vi "Generate Custom Error.vi"(8 "error in":errorcluster, 10 "PAR1":string, 11 "Enum":T1) -> (0 "error out":errorcluster)   [LabVIEW 2013, in "GOLPI library.lvlib"]
uses:
  GOLPI library.lvlib
  Custom Error Codes Enum Type Def.vi
  <vilib>/Utility/error.llb/Error Cluster From Error Code.vi
  <vilib>/ErrorRing/Error Ring.xnode
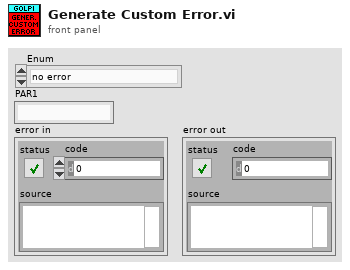
[diagram p1: front panel]
types:
  T1 = typedef "GOLPI library.lvlib/Custom Error Codes Enum Type Def.vi" = enum16{"no error", "00 working directory PAR1 missing", "01 octave binary PAR1 missing", "02 octave report error PAR1", "03 empty output last cmd PAR1", "04 missing temporary file PAR1", "10 var PAR1 not string", "11 var PAR1 not num, scal, ~compl", "12 var PAR1 not num, scal, compl", "13 var PAR1 not num, vect, ~compl", "14 var PAR1 not num, vect, compl", "15 var PAR1 not num, mat, ~compl", "16 var PAR1 not num, mat, ~compl", "99 not finished"}
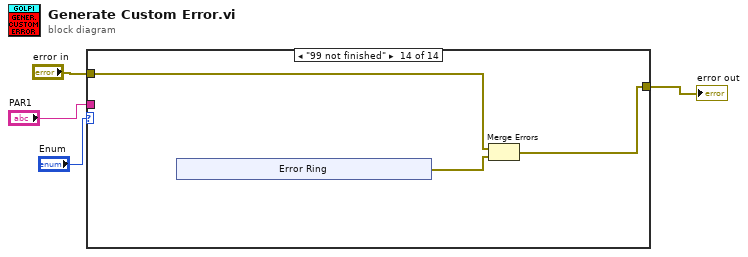
[diagram p0: block diagram]
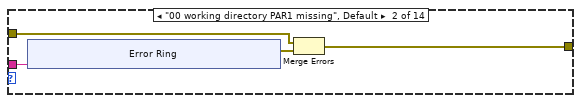
[diagram p3: hidden frame]
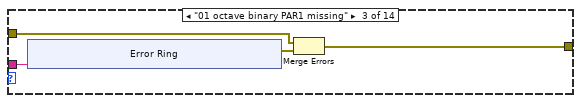
[diagram p4: hidden frame]
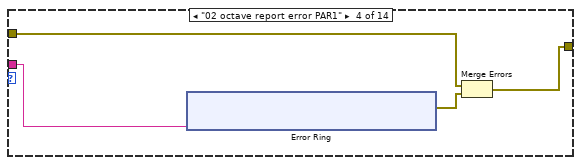
[diagram p5: hidden frame]
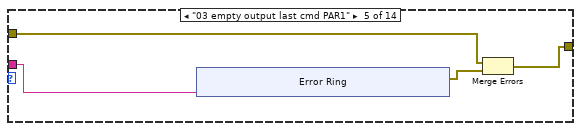
[diagram p6: hidden frame]
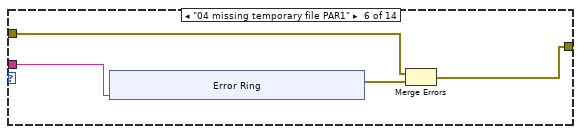
[diagram p7: hidden frame]
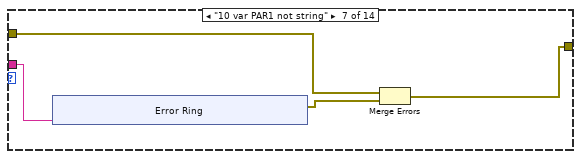
[diagram p8: hidden frame]
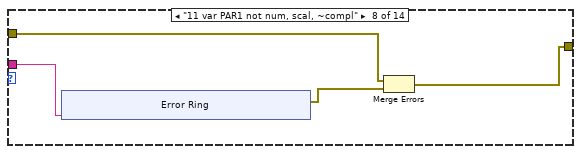
[diagram p9: hidden frame]
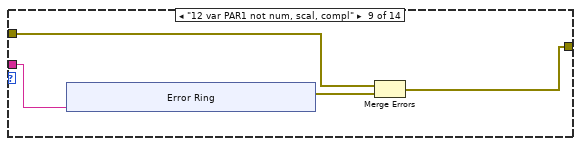
[diagram p10: hidden frame]
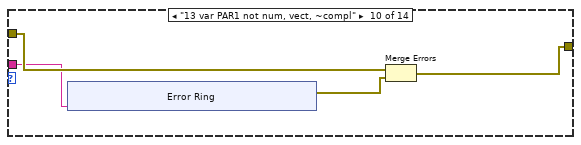
[diagram p11: hidden frame]
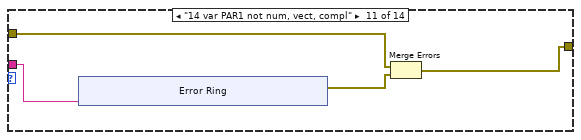
[diagram p12: hidden frame]
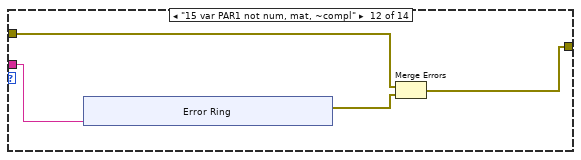
[diagram p13: hidden frame]
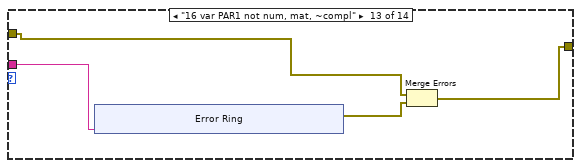
[diagram p14: hidden frame]
diagram:
  n1 = case shown="\"99 not finished\"" "Enum" {
    tunnel: "PAR1" -> [_ w9 w20 w29 w42 w50 w61 w72 w84 w94 w106 w116 w127 _]
    tunnel: [w5 w7 w18 w28 w39 w51 w62 w73 w83 w96 w105 w117 w128 w138] -> w1
    tunnel: "error in" -> [w5 w6 w17 w30 w40 w52 w63 w74 w86 w97 w107 w118 w129 w139]
    frame "no error" {
    }
    frame "00 working directory PAR1 missing", Default {
      n2 = xnode "Error Ring"("parameter 0"=w9) -> ("error out"=w8:errorcluster)
      n3 = Merge Errors(w6, w8) -> (w7:errorcluster)
    }
    frame "01 octave binary PAR1 missing" {
      n4 = xnode "Error Ring"("parameter 0"=w20) -> ("error out"=w19:errorcluster)
      n5 = Merge Errors(w17, w19) -> (w18:errorcluster)
    }
    frame "02 octave report error PAR1" {
      n6 = xnode "Error Ring"("parameter 0"=w29) -> ("error out"=w31:errorcluster)
      n7 = Merge Errors(w30, w31) -> (w28:errorcluster)
    }
    frame "03 empty output last cmd PAR1" {
      n8 = xnode "Error Ring"("parameter 0"=w42) -> ("error out"=w41:errorcluster)
      n9 = Merge Errors(w40, w41) -> (w39:errorcluster)
    }
    frame "04 missing temporary file PAR1" {
      n10 = xnode "Error Ring"("parameter 0"=w50) -> ("error out"=w53:errorcluster)
      n11 = Merge Errors(w52, w53) -> (w51:errorcluster)
    }
    frame "10 var PAR1 not string" {
      n12 = xnode "Error Ring"("parameter 0"=w61) -> ("error out"=w64:errorcluster)
      n13 = Merge Errors(w63, w64) -> (w62:errorcluster)
    }
    frame "11 var PAR1 not num, scal, ~compl" {
      n14 = xnode "Error Ring"("parameter 0"=w72) -> ("error out"=w75:errorcluster)
      n15 = Merge Errors(w74, w75) -> (w73:errorcluster)
    }
    frame "12 var PAR1 not num, scal, compl" {
      n16 = xnode "Error Ring"("parameter 0"=w84) -> ("error out"=w85:errorcluster)
      n17 = Merge Errors(w86, w85) -> (w83:errorcluster)
    }
    frame "13 var PAR1 not num, vect, ~compl" {
      n18 = xnode "Error Ring"("parameter 0"=w94) -> ("error out"=w95:errorcluster)
      n19 = Merge Errors(w97, w95) -> (w96:errorcluster)
    }
    frame "14 var PAR1 not num, vect, compl" {
      n20 = xnode "Error Ring"("parameter 0"=w106) -> ("error out"=w108:errorcluster)
      n21 = Merge Errors(w107, w108) -> (w105:errorcluster)
    }
    frame "15 var PAR1 not num, mat, ~compl" {
      n22 = xnode "Error Ring"("parameter 0"=w116) -> ("error out"=w119:errorcluster)
      n23 = Merge Errors(w118, w119) -> (w117:errorcluster)
    }
    frame "16 var PAR1 not num, mat, ~compl" {
      n24 = xnode "Error Ring"("parameter 0"=w127) -> ("error out"=w130:errorcluster)
      n25 = Merge Errors(w129, w130) -> (w128:errorcluster)
    }
    frame "99 not finished" {
      n26 = xnode "Error Ring"() -> ("error out"=w140:errorcluster)
      n27 = Merge Errors(w139, w140) -> (w138:errorcluster)
    }
  }
  "error out" <- w1
